vi "GetArrayIndexFromCoordinate.vi"(8 "error in (no error)":errorcluster, 10 "Coords in":T1, 11 "Array in":refnum<vi>) -> (0 "error out":errorcluster, 1 "in element? (1D arrays only)":bool, 2 "Element Indexes":cluster{"Horizontal":u32, "Vertical":u32}, 3 "Array out":refnum<vi>, 4 "Position In array coords":T2, 6 "Relative Position in element":cluster{"Horizontal":u32, "Vertical":u32})   [LabVIEW 2023]
doc: "This VI gets an Icon array and mouse coordinates and returns the index of the array element at coordinates\nposition."
uses:
  <vilib>/Utility/miscctls.llb/LVPositionTypeDef.ctl
  <vilib>/Utility/miscctls.llb/LVPoint32TypeDef.ctl
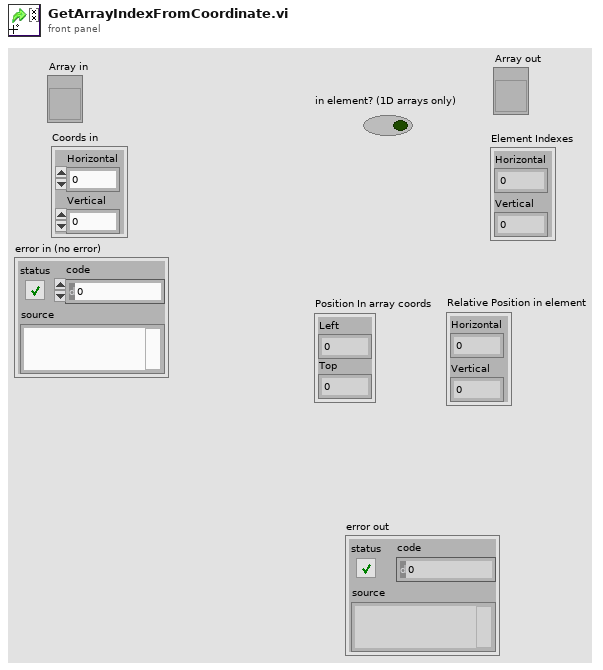
[diagram p1: front panel]
types:
  T1 = typedef "LVPoint32TypeDef.ctl" = cluster{"Horizontal":i32, "Vertical":i32}
  T2 = typedef "LVPositionTypeDef.ctl" = cluster{"Left":i32, "Top":i32}
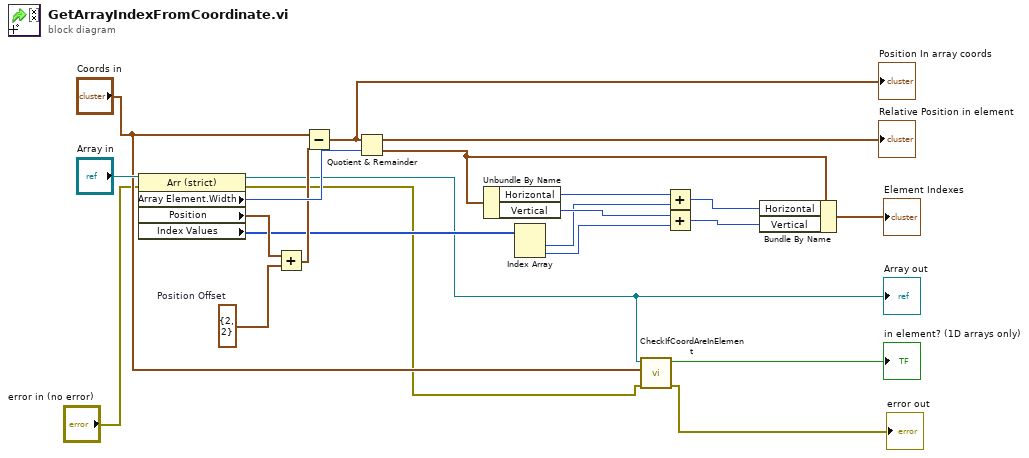
[diagram p0: block diagram]
diagram:
  w19 = T2 {"Left"=2, "Top"=2}  # Position Offset
  n1 = property on="Property Node" class="Arr (strict)"(reference="Array in", error in="error in (no error)") -> (reference out=w10:refnum<vi>, error out=w2:errorcluster, "Array Element.Width"=w22:u32, "Position"=w17:T2, "Index Values"=w16:u32[])
  "Array out" <- w10
  n2 = Add(x=w17, y=w19) -> (x+y=w20:T2)
  n3 = Subtract(x="Coords in", y=w20) -> (x-y=w4:T1)
  "Position In array coords" <- w4
  n4 = Quotient & Remainder(x=w4, y=w22) -> (x-y*floor(x/y)=→"Relative Position in element":cluster{"Horizontal":u32, "Vertical":u32}, floor(x/y)=w8:cluster{"Horizontal":u32, "Vertical":u32})
  n5 = Unbundle By Name(w8) -> ("Horizontal"=w15:u32, "Vertical"=w14:u32)
  n6 = Index Array(array=w16) -> (element #1=w12:u32, element #2=w13:u32)  [unwired: 2 in]
  n7 = call "CheckIfCoordAreInElement.vi"("error in (no error)"=w2, "Coords"="Coords in", "Array in"=w10) -> ("error out"=→"error out":errorcluster, "in element?"=→"in element? (1D arrays only)":bool)  [unwired: 7 in]
  n8 = Add(x=w15, y=w12) -> (x+y=w7:u32)
  n9 = Add(x=w14, y=w13) -> (x+y=w6:u32)
  n10 = Bundle By Name(cluster=w8, "Horizontal"=w7, "Vertical"=w6) -> (→"Element Indexes":cluster{"Horizontal":u32, "Vertical":u32})
